vi "Test set cell value.vi"(11 "Test Case In":refnum<class "Test Cases.lvclass">) -> (0 "error out":errorcluster, 3 "Test Case Out":refnum<class "Test Cases.lvclass">)   [LabVIEW 2024, in "Test Cases.lvclass"]
uses:
  Test Cases.lvclass
  C:/Program Files/National Instruments/LabVIEW 2025/vi.lib/Astemes/LUnit/Test Case.lvclass
  source/Grid/SourceGrid.lvclass
  source/Cells/Check Box/Check Box.lvclass
  D:/git/Sourcegrid-LabVIEW/source/Cells/Cell/Cell.lvclass
  <vilib>/Astemes/LUnit/Test Case.lvclass/Test Case.ctl
  Test Cases.lvclass/Test Cases.ctl
  <vilib>/Astemes/LUnit/Test Case.lvclass
  D:/git/Sourcegrid-LabVIEW/dll/SourceGrid.dll
  dll/SourceGrid.dll
panel:
  in  "stop":bool
  in  "Grid Container":refnum<k24>(container)
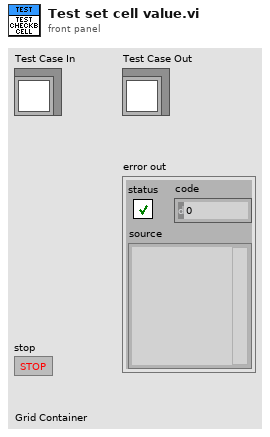
[diagram p1: front panel]
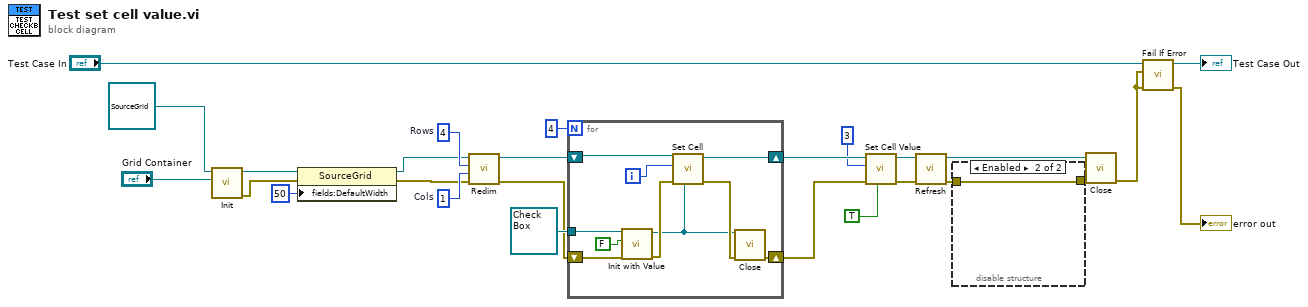
[diagram p0: block diagram]
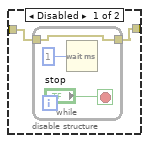
[diagram p2: hidden frame]
diagram:
  w22 = 1  # Cols
  w23 = 4  # Rows
  n1 = call-dynamic "Init.vi"("Sourcegrid Container"="Grid Container", "Grid in"=refnum<class "SourceGrid.lvclass"> refnum) -> ("error out"=w11:errorcluster, "Grid out"=w19:refnum<class "SourceGrid.lvclass">)  [unwired: 8 in]
  n2 = property class="SourceGrid"(reference=w19, error in=w11, "fields:DefaultWidth"=50 ("DefaultWidth")) -> (reference out=w18:refnum<class "SourceGrid.lvclass">, error out=w17:errorcluster)
  n3 = call "Redim.vi"("error in"=w17, "Columns"=w22, "Rows"=w23, "Sourcegrid in"=w18) -> ("error out"=w6:errorcluster, "Sourcegrid out"=w15:refnum<class "SourceGrid.lvclass">)  [unwired: 6 in]
  n4 = for {
    N: 4 -> [_]
    shift-right: [w34] -> w7
    shift-left: w6 -> [w31]
    shift-right: [w36] -> w4
    shift-left: w15 -> [w35]
    tunnel: refnum<class "Check Box.lvclass"> refnum ("Cell in") -> [w32]
    i -> [w30]
    n5 = call-dynamic "Init with Value.vi"("error in"=w31, "Value"=FALSE, "Check Box in"=w32) -> ("error out"=w29:errorcluster, "Check Box out"=w27:refnum<class "Check Box.lvclass">)  [unwired: 7 in]
    n6 = call "Set Cell.vi"("Cell"=w27, "error in"=w29, "Row"=w30, "Sourcegrid in"=w35) -> ("error out"=w33:errorcluster, "Sourcegrid out"=w36:refnum<class "SourceGrid.lvclass">)  [unwired: 6 in]
    n7 = call-dynamic "Close.vi"("error in"=w33, "Cell in"=w27) -> ("error out"=w34:errorcluster)  [unwired: 8 in, 1 out]
  }
  n8 = call "Set Cell Value.vi"("Value"=TRUE, "error in"=w7, "Row"=3, "SourceGrid in"=w4) -> ("error out"=w5:errorcluster, "SourceGrid out"=w3:refnum<class "SourceGrid.lvclass">)  [unwired: 6 in]
  n9 = call "Refresh.vi"("error in"=w5, "SourceGrid in"=w3) -> ("error out"=w9:errorcluster, "SourceGrid out"=w13:refnum<class "SourceGrid.lvclass">)  [unwired: 8 in]
  n10 = disable-structure shown="Enabled" {
    disable-tunnel: w9 -> [w38 w42]
    disable-tunnel: [w37 w42] -> w8
    frame Disabled {
      n11 = while {
        tunnel: w38 -> [w39]
        tunnel: [w39] -> w37
        stop <- "stop" stop-if-true
        n12 = Wait (ms)(milliseconds to wait=u32 1) -> ()  [unwired: 1 out]
      }
    }
    frame Enabled {
    }
  }
  n13 = call-dynamic "Close.vi"("error in"=w8, "Sourcegrid in"=w13) -> ("error out"=w21:errorcluster)  [unwired: 8 in, 1 out]
  n14 = call <vilib>:"Fail If Error.vi"("error in (no error)"=w21, "Assert error"=w21, "LUnit Test Case In"="Test Case In") -> ("error out"=→"error out":errorcluster, "LUnit Test Case Out"=→"Test Case Out":refnum<class "Test Cases.lvclass">)  [unwired: 7 in]
